vi "SN_coords_precess.vi"() -> ()   [LabVIEW 2010]
panel:
  out "DEC (J2KSN)":dbl format="%<%H:%M:%S%3u>t"
  out "RA (J2KSN)":dbl format="%<%H:%M:%S%3u>t"
  out "EquatorialSystem":i32(ring) items=["equOther", "equLocalTopocentric", "equJ2000", "equJ2050", "equB1950"]
  out "DEC (J2000)":dbl format="%<%H:%M:%S%3u>t"
  out "RA (J2000)":dbl format="%<%H:%M:%S%3u>t"
  out "DEC (JNOW)":dbl format="%<%H:%M:%S%3u>t"
  out "RA (JNOW)":dbl format="%<%H:%M:%S%3u>t"
  in  "ScopeSim._Telescope":refnum<k7>
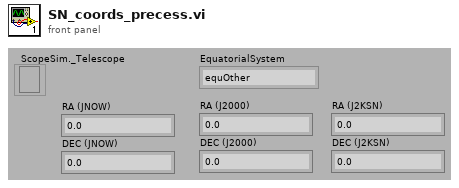
[diagram p1: front panel]
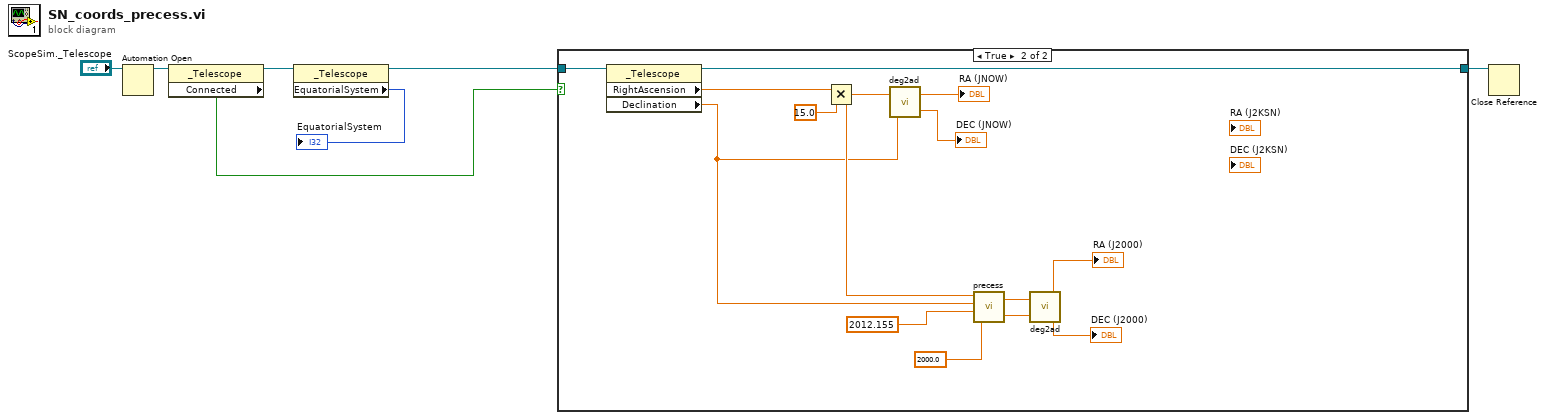
[diagram p0: block diagram]
diagram:
  n1 = Automation Open(Automation Refnum="ScopeSim._Telescope") -> (Automation Refnum=w6:refnum<k7>)  [unwired: 3 in, 1 out]
  n2 = property class="_Telescope"(reference=w6) -> (reference out=w3:refnum<k7>, "Connected"=w1:bool)  [unwired: 1 in, 1 out]
  n3 = property class="_Telescope"(reference=w3) -> (reference out=w2:refnum<k7>, "EquatorialSystem"=→"EquatorialSystem":i32)  [unwired: 1 in, 1 out]
  n4 = case shown="True" w1 {
    tunnel: w2 -> [w8 w22]
    tunnel: [w8 w20] -> w5
    frame False {
    }
    frame True {
      n5 = property class="_Telescope"(reference=w22) -> (reference out=w20:refnum<k7>, "RightAscension"=w13:dbl, "Declination"=w11:dbl)  [unwired: 1 in, 1 out]
      n6 = Multiply(x=w13, y=15.0) -> (x*y=w12:dbl)
      n7 = call "deg2ad.vi"("DEC (°)"=w11, "RA (°)"=w12) -> ("DEC (sec)"=→"DEC (JNOW)":dbl, "RA (sec)"=→"RA (JNOW)":dbl)
      n8 = call "precess.vi"("Eq2"=2000.0 ("Eq1"), "Eq1"=2012.155, "DEC 1"=w11, "RA 1"=w12) -> ("DEC 2"=w16:dbl, "RA 2"=w17:dbl)
      n9 = call "deg2ad.vi"("DEC (°)"=w16, "RA (°)"=w17) -> ("DEC (sec)"=→"DEC (J2000)":dbl, "RA (sec)"=→"RA (J2000)":dbl)
    }
  }
  n10 = Close Reference(reference=w5) -> ()  [unwired: 1 in, 1 out]
